vi "LVClasse_Intensity ctor from HasoSlopes.vi"(0 "Intensity in":refnum<class "Intensity.lvclass">, 5 "HasoSlopes":refnum<class "HasoSlopes.lvclass">, 11 "error in (no error)":errorcluster) -> (4 "Intensity out":refnum<class "Intensity.lvclass">, 15 "error out":errorcluster)   [LabVIEW 2020, in "Intensity.lvclass"]
uses:
  Intensity.lvclass
  HasoSlopes.lvclass
  Handle creation.ctl
  Intensity.lvclass/Intensity.ctl
  LVClass_HasoSlopes Read HasoSlopes _ property.vi
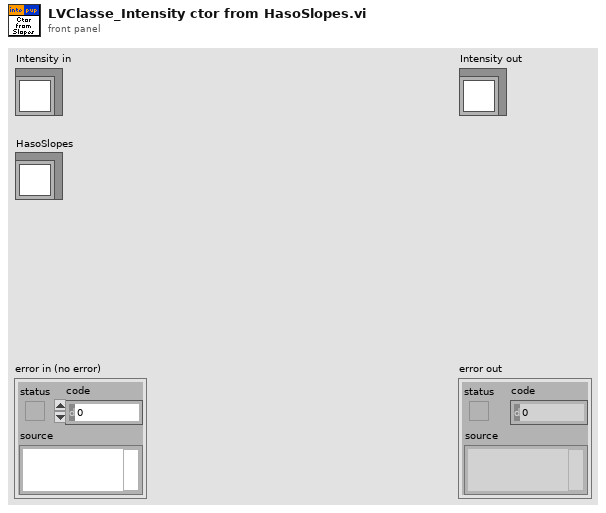
[diagram p1: front panel]
types:
  T1 = typedef "Handle creation.ctl" = enum16{"By ctor", "By write function"}
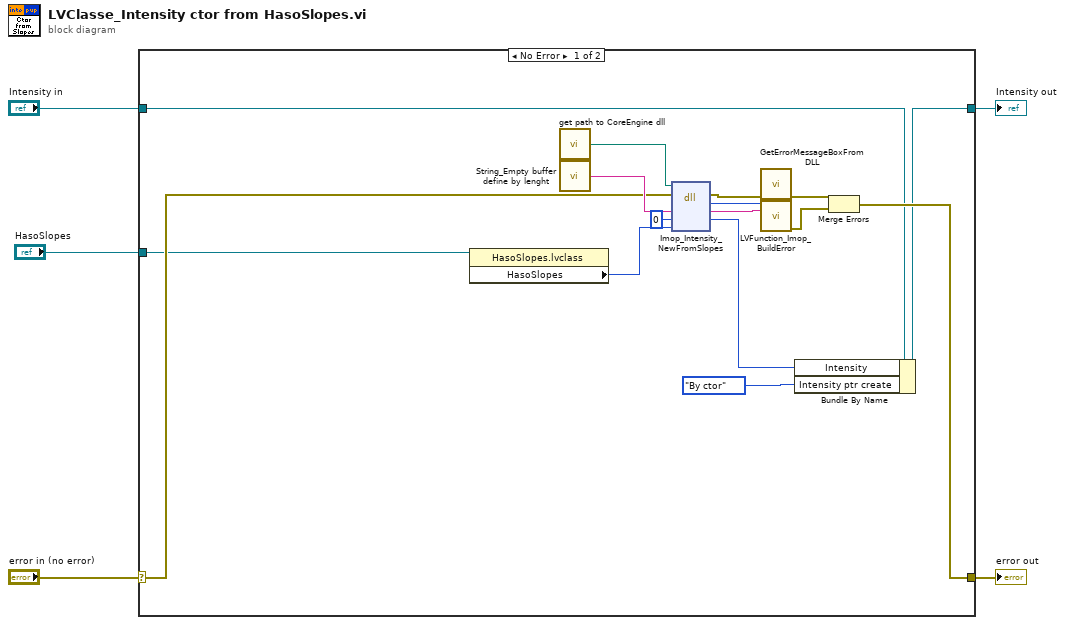
[diagram p0: block diagram]
diagram:
  n1 = case shown="No Error" "error in (no error)" {
    selector: "error in (no error)" -> [w14 w23]
    tunnel: [w13 w23] -> w4
    tunnel: [w9 w22] -> w2
    tunnel: "Intensity in" -> [w10 w22]
    tunnel: "HasoSlopes" -> [w12 _]
    frame No Error {
      n2 = property class="HasoSlopes.lvclass"(reference=w12) -> ("HasoSlopes"=w11:i32)  [unwired: 1 in, 2 out]
      n3 = call "get path to CoreEngine dll.vi"() -> ("path to c_interface_vc100.dll"=w18:path)  [unwired: 12 in, 3 out]
      n4 = call "String_Empty buffer define by lenght.vi"() -> ("Empty buffer"=w19:string)  [unwired: 1 in]
      n5 = dll-call lib="D:/FLE/0.Code/CoreEngine4_Suite/LV2011_interface/DLLs/c_interface_vc100.dll" fn="Imop_Intensity_NewFromSlopes"(path in=w18, error in=w14, "message"=w19, "Intensity"=0 ("Phase"), "HasoSlopes"=w11) -> (error out=w17:errorcluster, "return type"=w21:i32, "message"=w20:string, "Intensity"=w8:i32)  [unwired: 2 in, 1 out]
      n6 = call "GetErrorMessageBoxFromDLL.vi"("error IN"=w17) -> ("error OUT"=w16:errorcluster)  [unwired: 10 in]
      n7 = call "LVFunction_Imop_BuildError.vi"("code"=w21, "String to Prepend to source (\"\")"=w20) -> ("error out"=w15:errorcluster)  [unwired: 13 in]
      n8 = Bundle By Name(cluster=w10, "Intensity"=w8, "Intensity ptr create"=Handle_creation."By ctor" ("Phase ptr create")) -> (w9:refnum<class "Intensity.lvclass">)
      n9 = Merge Errors(w16, w15) -> (w13:errorcluster)
    }
    frame Error {
    }
  }
  "error out" <- w4
  "Intensity out" <- w2
